vi "DAQ.TimedLoop2.vi"(8 "error in (no error)":errorcluster, 11 "Instrument.DAQ in":refnum<class "Instrument.DAQ.lvclass">) -> (0 "error out":errorcluster, 3 "Instrument.DAQ out":refnum<class "Instrument.DAQ.lvclass">)   [LabVIEW 2019]
uses:
  Instrument.DAQ.lvclass
  Typedefs/Set State-enum.ctl
  <vilib>/JKI/JKI SMO/SMO/SMO.lvclass
  C:/Program Files/National Instruments/LabVIEW 2019/vi.lib/JKI/JKI SMO/SMO/SMO.lvclass
panel:
  # "!!!!!!!!!!!!!!!!!!!!!!!!!!!!!!!!!!!!!!!!!!!!!!!!!!!!!!!!!!!!!!!!!!!!!!!!\nTHIS IS AN EXPERIMENTAL BLOCKING CALL TO:\nGenerate\nRead/Write\nDSP\nIt should listen to events that change AO or REF Channels.\nInside there is a timed loop that will not stop unless it receives events for Set State = stop; SMO Stop; or SMO error\n!!!!!!!!!!!!!!!!!!!!!!!!!!!!!!!!!!!!!!!!!!!!!!!!!!!!!!!!!!!!!!!!!!!!!"
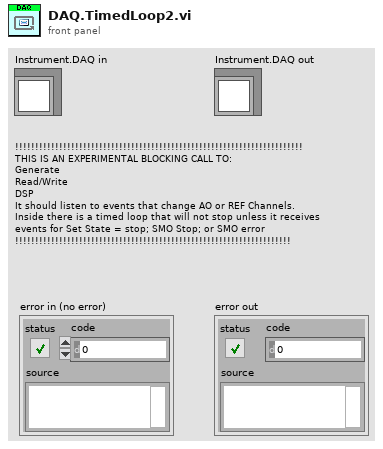
[diagram p1: front panel]
types:
  T1 = typedef "SMO.lvclass/Protected Events.ctl" = cluster{"StopProcesses":refnum<user-event>, "AbortProcesses":refnum<user-event>, "Config Changed":refnum<user-event>, "Dependency":refnum<user-event>}
  T2 = typedef "Instrument.Lockin.lvlib/Instrument.DAQ.lvclass/PrivateEvents--Cluster.ctl" = cluster{"setAOconfig":refnum<user-event>, "setAIconfig":refnum<user-event>, "setAO":refnum<user-event>, "setREF":refnum<user-event>, "setSampling":refnum<user-event>, "setState":refnum<user-event>, "setInputGain":refnum<user-event>, "setOutputGain":refnum<user-event>, "setSweep":refnum<user-event>, "measureOffset":refnum<user-event>, "zeroOffset":refnum<user-event>, "setPreFilter":refnum<user-event>, "autoConfigureDAQ":refnum<user-event>, "setCalibration":refnum<user-event>, "setAI":refnum<user-event>, "zeroPhase":refnum<user-event>, "setAmplitudeLimit":refnum<user-event>, "setLinkFrequencies":refnum<user-event>, "showUI":refnum<user-event>, "setInputOffset":refnum<user-event>, "setDCLimit":refnum<user-event>}
  T3 = typedef "Instrument.Lockin.lvlib/Instrument.DAQ.lvclass/Set State-enum.ctl" = enum16{"start", "stop", "reset", "start sweep", "stop sweep"}
  T4 = typedef "Instrument.Lockin.lvlib/Instrument.DAQ.lvclass/Queue and Notifier.ctl" = cluster{"Message":refnum<queue>, "Stop":refnum<notifier>}
  T5 = typedef "Instrument.Lockin.lvlib/Instrument.DAQ.lvclass/AO.Channel--Cluster--Array.ctl" = T6[]
  T6 = typedef "Instrument.Lockin.lvlib/Instrument.DAQ.lvclass/AO.Channel--Cluster.ctl" = cluster{"Enable?":bool, "Channel":i32, "Amplitude":dbl, "Offset":dbl, "Frequency":dbl, "Phase":dbl, "Function":T7, "Sweeping?":bool, "Limit AC":bool, "Limit DC?":bool}
  T7 = typedef "Instrument.Lockin.lvlib/Instrument.DAQ.lvclass/AO.Channel.Function--Enum.ctl" = enum16{"Sine", "Triangle", "Square"}
  T8 = typedef "Instrument.Lockin.lvlib/Instrument.DAQ.lvclass/REF.Channel--Cluster--Array.ctl" = T9[]
  T9 = typedef "Instrument.Lockin.lvlib/Instrument.DAQ.lvclass/REF.Channel--Cluster.ctl" = cluster{"Enable?":bool, "Channel":i32, "Frequency":dbl, "Phase":dbl, "TC":dbl, "Roll-Off":i32}
  T10 = typedef "Instrument.Lockin.lvlib/Instrument.DAQ.lvclass/Results--Cluster.ctl" = cluster{"Time Stamp":timestamp, "Results (Dictionary)":cluster{"key":string, "value":dbl}[]}
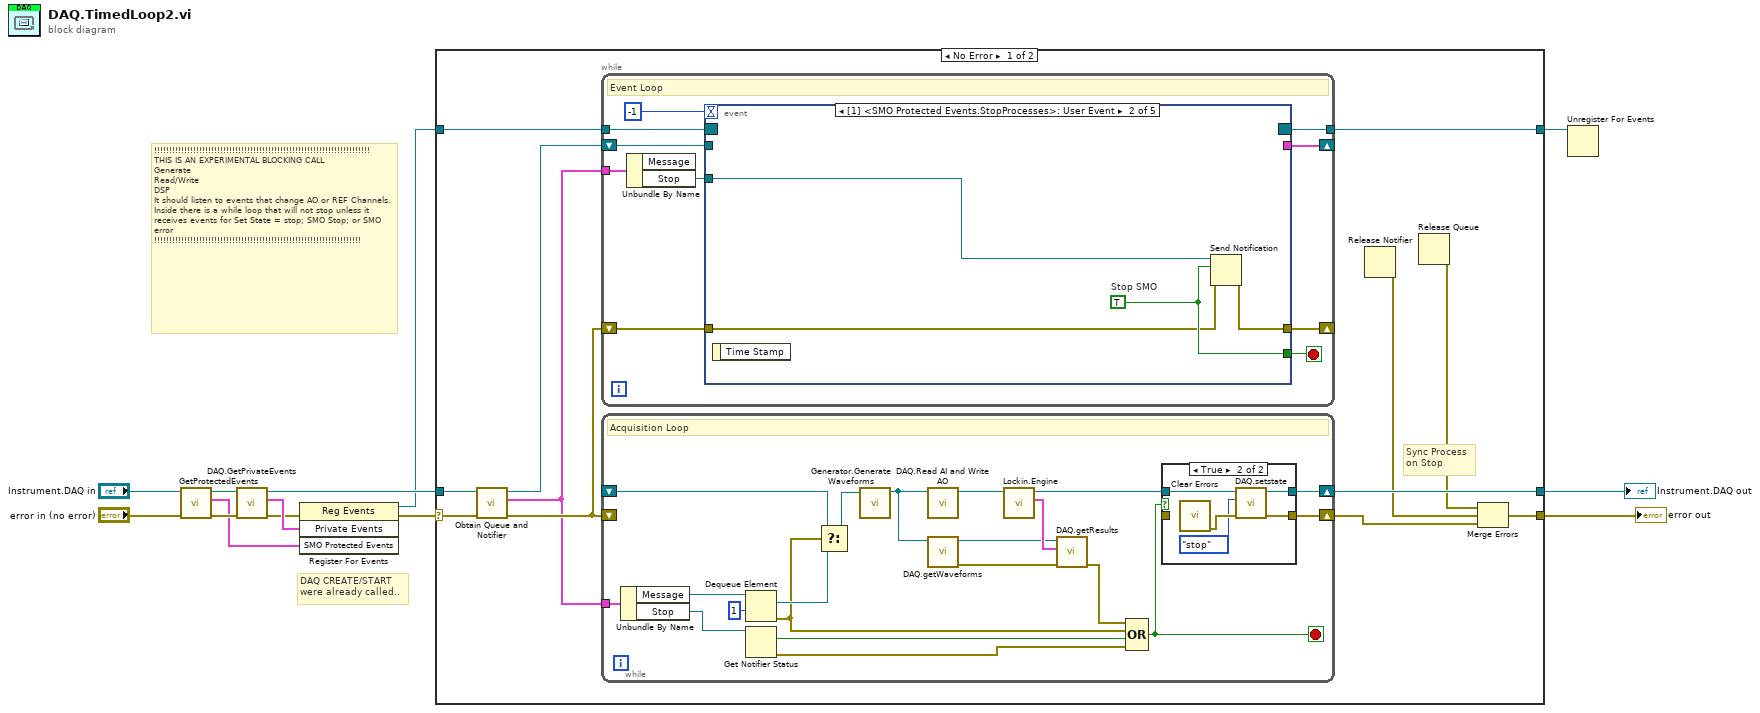
[diagram p0: block diagram]
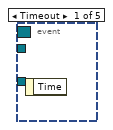
[diagram p3: hidden frame]
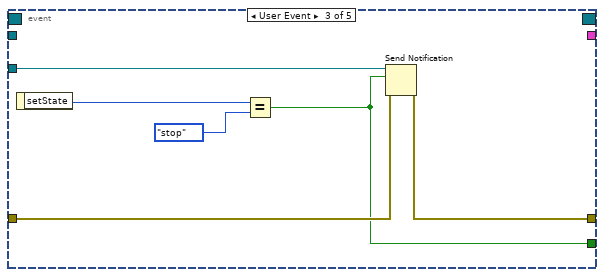
[diagram p4: hidden frame]
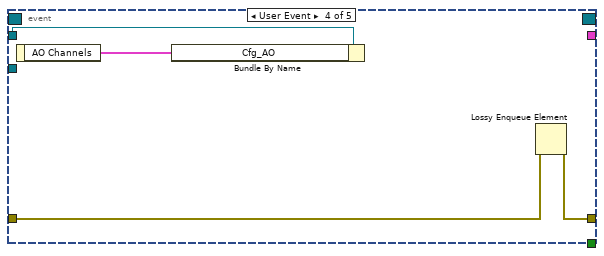
[diagram p5: hidden frame]
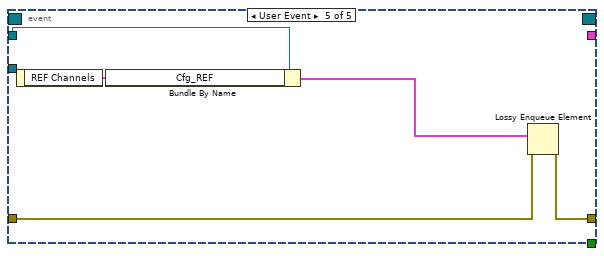
[diagram p6: hidden frame]
diagram:
  # "DAQ CREATE/START\nwere already called.."
  # "!!!!!!!!!!!!!!!!!!!!!!!!!!!!!!!!!!!!!!!!!!!!!!!!!!!!!!!!!!!!!!!!!!!!!!!!\nTHIS IS AN EXPERIMENTAL BLOCKING CALL\nGenerate\nRead/Write\nDSP\nIt should listen to events that change AO or REF Channels.\nInside there is a while loop that will not stop unless it receives events for Set State = stop; SMO Stop; or SMO error\n!!!!!!!!!!!!!!!!!!!!!!!!!!!!!!!!!!!!!!!!!!!!!!!!!!!!!!!!!!!!!!!!!!!!!"
  n1 = call <vilib>:"GetProtectedEvents.vi"("error in (no error)"="error in (no error)", "SMO"="Instrument.DAQ in") -> ("error out"=w6:errorcluster, "SMO Protected Events"=w5:T1, "SMO out"=w7:refnum<class "Instrument.DAQ.lvclass">)  [unwired: 7 in]
  n2 = call "DAQ.GetPrivateEvents.vi"("error in (no error)"=w6, "Instrument.DAQ"=w7) -> ("error out"=w2:errorcluster, "Private Events"=w4:T2, "Instrument.DAQ"=w3:refnum<class "Instrument.DAQ.lvclass">)  [unwired: 7 in]
  n3 = register-events(error in=w2, w4, w5) -> (reference out=w1:refnum<event-registration>, error out=w9:errorcluster)  [unwired: 1 in]
  n4 = case shown="No Error" w9 {
    selector: w9 -> [w17 w85]
    tunnel: w3 -> [w18 w86]
    tunnel: w1 -> [w25 w87]
    tunnel: [w23 w85] -> w10
    tunnel: [w24 w87] -> w8
    tunnel: [w22 w86] -> w12
    frame No Error {
      # "Sync Process\non Stop"
      n5 = call "Obtain Queue and Notifier.vi"("error in (no error)"=w17, "Instrument.DAQ in"=w18) -> ("error out"=w16:errorcluster, "Queue and Notifier"=w15:T4, "Instrument.DAQ"=w14:refnum<class "Instrument.DAQ.lvclass">)  [unwired: 7 in]
      n6 = while {
        tunnel: w25 -> [w62]
        tunnel: [w61] -> w24
        shift-right: [w55] -> _
        shift-left: w14 -> [w59]
        tunnel: w15 -> [w54]
        shift-right: [w57] -> _
        shift-left: w16 -> [w58]
        stop <- w60 stop-if-true
        # "Event Loop"
        n7 = Unbundle By Name(w54) -> ("Stop"=w53:refnum<notifier>)  [unwired: 1 out]
        n8 = event shown="[1] <SMO Protected Events.StopProcesses>: User Event" {
          selector: w62 -> [_ _ _ _ _]
          dyn-events: [_ _ _ _ _] -> w61
          timeout: -1 -> [_ _ _ _ _]
          tunnel: [_ w68 w71 _ _] -> w60
          tunnel: [_ w65 w69 w79 w84] -> w57
          tunnel: w59 -> [w63 w67 w75 w76 w83]
          tunnel: w58 -> [_ w66 w74 w77 w81]
          tunnel: [_ _ _ _ _] -> w55
          tunnel: w53 -> [_ w64 w70 _ _]
          event Timeout {
            n9 = event-data() -> ()  [unwired: 1 in, 1 out]
          }
          event User Event {
            w68 = TRUE  # Stop SMO
            n10 = event-data() -> ()  [unwired: 1 in, 1 out]
            n11 = Send Notification(notification=w68, notifier=w64, error in (no error)=w66) -> (error out=w65:errorcluster)  [unwired: 1 out]
          }
          event User Event {
            n12 = event-data() -> ("setState"=w73:T3)  [unwired: 1 in]
            n13 = Equal?(x=w73, y=Set_State-enum."stop") -> (x = y?=w71:bool)
            n14 = Send Notification(notification=w71, notifier=w70, error in (no error)=w74) -> (error out=w69:errorcluster)  [unwired: 1 out]
          }
          event User Event {
            n15 = event-data() -> ("AO Channels"=w78:T5)  [unwired: 1 in]
            n16 = Bundle By Name(cluster=w76, "Cfg_AO"=w78) -> ()  [unwired: 1 out]
            n17 = Lossy Enqueue Element(error in (no error)=w77) -> (error out=w79:errorcluster)  [unwired: 2 in, 3 out]
          }
          event User Event {
            n18 = event-data() -> ("REF Channels"=w82:T8)  [unwired: 1 in]
            n19 = Bundle By Name(cluster=w83, "Cfg_REF"=w82) -> (w80:cluster{})
            n20 = Lossy Enqueue Element(element=w80, error in (no error)=w81) -> (error out=w84:errorcluster)  [unwired: 1 in, 3 out]
          }
        }
      }
      n21 = while {
        tunnel: w15 -> [w28]
        shift-right: [w38] -> w22
        shift-left: _ -> [w32]
        shift-right: [w37] -> w21
        shift-left: w16 -> [_]
        stop <- w40 stop-if-true
        # "Acquisition Loop"
        n22 = Unbundle By Name(w28) -> ("Message"=w27:refnum<queue>, "Stop"=w26:refnum<notifier>)
        n23 = Dequeue Element(queue=w27, timeout in ms (-1)=1) -> (element=w33:refnum<class "Instrument.DAQ.lvclass">, error out=w30:errorcluster)  [unwired: 1 in, 2 out]
        n24 = Get Notifier Status(notifier=w26) -> (current notification=w45:bool, error out=w44:errorcluster)  [unwired: 1 in, 3 out]
        n25 = Select(t=w32, s=w30, f=w33) -> (s? t:f=w31:refnum<class "Instrument.DAQ.lvclass">)
        n26 = call "Generator.Generate Waveforms.vi"("Instrument.DAQ"=w31) -> ("Instrument.DAQ"=w36:refnum<class "Instrument.DAQ.lvclass">)  [unwired: 9 in, 1 out]
        n27 = call "DAQ.Read AI and Write AO.vi"("Instrument.DAQ in"=w36) -> ("Instrument.DAQ out"=w43:refnum<class "Instrument.DAQ.lvclass">)  [unwired: 9 in, 1 out]
        n28 = call "DAQ.getWaveforms.vi"("Instrument.DAQ"=w36) -> ("error out"=w35:errorcluster, "Instrument.DAQ"=w34:refnum<class "Instrument.DAQ.lvclass">)  [unwired: 9 in]
        n29 = call "Lockin.Engine.vi"("Instrument.DAQ"=w43) -> ("<Results> (X,Y,R,Theta,Mean)"=w42:T10, "Instrument.DAQ out"=w39:refnum<class "Instrument.DAQ.lvclass">)  [unwired: 8 in, 1 out]
        n30 = call "DAQ.getResults.vi"("error in (no error)"=w35, "Results"=w42, "Instrument.DAQ"=w34) -> ("error out"=w29:errorcluster)  [unwired: 7 in, 1 out]
        n31 = Compound Arithmetic op=OR(w29, w30, w45, w44) -> (w40:bool)
        n32 = case shown="True" w40 {
          tunnel: w39 -> [w46 w52]
          tunnel: [w46 w51] -> w38
          tunnel: [w47 w50] -> w37
          tunnel: _ -> [w47 _]
          frame False {
          }
          frame True {
            n33 = call <vilib>:"Clear Errors.vi"() -> ("error out"=w49:errorcluster)  [unwired: 6 in, 1 out]
            n34 = call "DAQ.setstate.vi"("error in (no error)"=w49, "setState"=Set_State-enum."stop", "Instrument.DAQ"=w52) -> ("error out"=w50:errorcluster, "Instrument.DAQ out"=w51:refnum<class "Instrument.DAQ.lvclass">)  [unwired: 7 in]
          }
        }
      }
      n35 = Release Notifier() -> (error out=w20:errorcluster)  [unwired: 3 in, 2 out]
      n36 = Release Queue() -> (error out=w19:errorcluster)  [unwired: 3 in, 2 out]
      n37 = Merge Errors(w19, w20, w21) -> (w23:errorcluster)
    }
    frame Error {
    }
  }
  "Instrument.DAQ out" <- w12
  "error out" <- w10
  n38 = Unregister For Events(event registration refnum=w8) -> ()  [unwired: 1 in, 1 out]
